vi "Msg Not In Unified Msgs--error.vi"() -> (2 "Error":errorcluster)   [LabVIEW 2020, in "jettl.lvlib"]
uses:
  jettl.lvlib
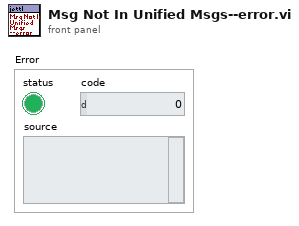
[diagram p1: front panel]
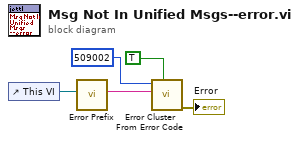
[diagram p0: block diagram]
diagram:
  n1 = control-ref of="This VI"() -> (w4:refnum<vi>)
  n2 = call "Error Prefix.vi"("VI Ref"=w4) -> ("Prefix"=w3:string)  [unwired: 10 in]
  n3 = call <vilib>:"Error Cluster From Error Code.vi"("show call chain? (False)"=TRUE, "error message (\"\")"=w3, "error code (0)"=509002) -> ("error out"=→"Error":errorcluster)  [unwired: 6 in]
